vi "Set Running.vi"(8 "error in (no error)":errorcluster, 10 "Running":bool, 11 "Panel in":refnum<class "Panel.lvclass">) -> (0 "error out":errorcluster, 3 "Panel out":refnum<class "Panel.lvclass">)   [LabVIEW 2018, in "OOPanel.lvlib" / "Panel.lvclass"]
uses:
  Panel.lvclass
  Panel.lvclass/Panel.ctl
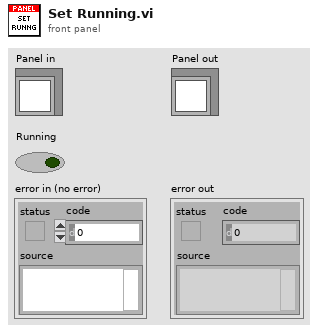
[diagram p1: front panel]
types:
  T1 = typedef "OOPanel.lvlib/Panel.lvclass/Ref Data.ctl" = cluster{"Panel VI":refnum<vi>, "Close":bool, "Panel Events":T2, "Running":bool, "Desired Size":T3, "Subpanel":refnum<vi>, "State":T4}
  T2 = typedef "OOPanel.lvlib/Panel.lvclass/Panel Events.ctl" = cluster{"Close":refnum<user-event>, "Visibility Changed":refnum<user-event>}
  T3 = typedef "OOPanel.lvlib/Panel.lvclass/Desired Size.ctl" = cluster{"Width":i16, "Height":i16}
  T4 = typedef "OOPanel.lvlib/Panel.lvclass/State.ctl" = enum16{"Idle", "Hidden", "Visible", "Subpanel"}
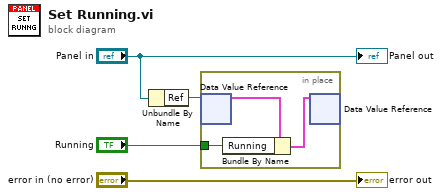
[diagram p0: block diagram]
diagram:
  n1 = Unbundle By Name("Panel in") -> ("Ref"=w2:refnum<data-value>)
  n2 = in-place {
    in-place-border: "Running" -> [w6]
    n3 = in-place-dvr #1(w2) -> (w7:T1)  [unwired: 1 out]
    n4 = Bundle By Name(cluster=w7, "Running"=w6) -> (w5:T1)
    n5 = in-place-dvr #1(w5) -> ()  [unwired: 2 out]
  }
  "error out" <- "error in (no error)"
  "Panel out" <- "Panel in"
